vi "ROI_transform_self.vi"(6 "Color":u32[](array[colorbox])=[16860], 9 "extrinsic":cluster{"extrinsic":dbl[][], i32[]}, 10 "ROI discriptor":T2, 11 "Refnum in":T1) -> (3 "Image Out":T1)   [LabVIEW 2017]
uses:
  <vilib>/vision/Image Controls.llb/IMAQ Image.ctl
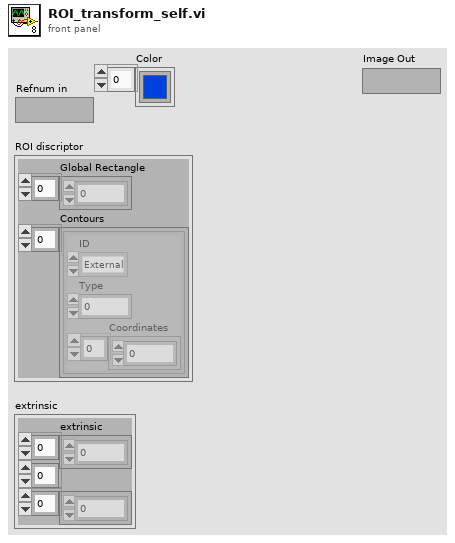
[diagram p1: front panel]
types:
  T1 = typedef "IMAQ Image.ctl" = refnum<image>
  T2 = cluster{"Global Rectangle":i32[], "Contours":cluster{"ID":enum32{"External", "Internal"}, "Type":u32, "Coordinates":i32[]}[]}
  T3 = cluster{"Start Point":cluster{"X":i32, "Y":i32}}[][]
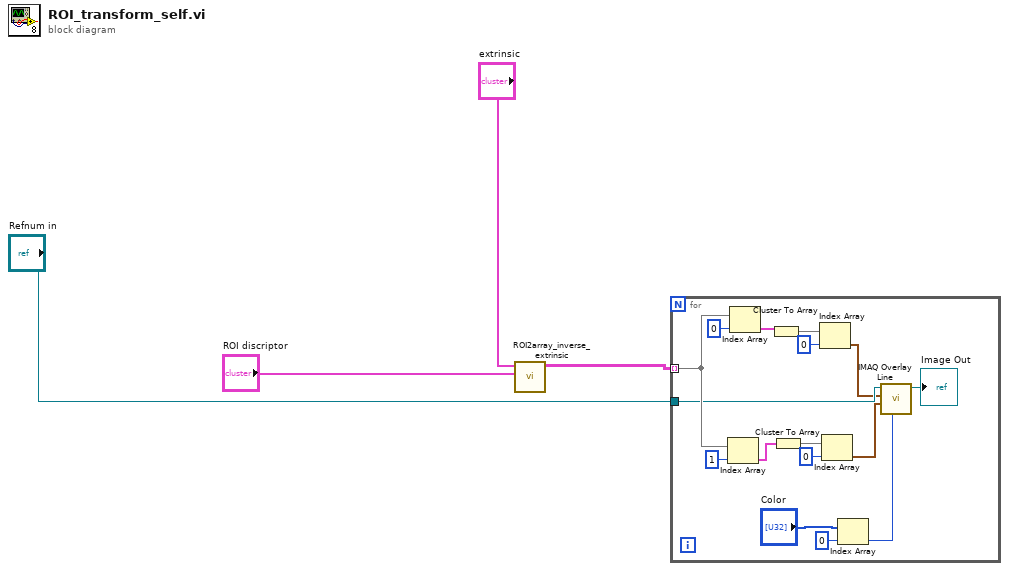
[diagram p0: block diagram]
diagram:
  n1 = call "ROI2array_inverse_extrinsic.vi"("Pad ROI 1"="ROI discriptor", "Cluster"="extrinsic") -> ("Array"=w2:T3)  [unwired: 9 in]
  n2 = for {
    tunnel: "Refnum in" -> [w14]
    tunnel: w2 -> [w19] mode=indexing
    n3 = Index Array(array=w19, index=1) -> (element=w10:cluster{"Start Point":cluster{"X":i32, "Y":i32}})
    n4 = Index Array(array=w19, index=0) -> (element=w17:cluster{"Start Point":cluster{"X":i32, "Y":i32}})
    n5 = Cluster To Array(cluster=w17) -> (array=w15:cluster{"X":i32, "Y":i32}[])
    n6 = Cluster To Array(cluster=w10) -> (array=w12:cluster{"X":i32, "Y":i32}[])
    n7 = Index Array(array=w15, index=0) -> (element=w13:cluster{"X":i32, "Y":i32})
    n8 = Index Array(array=w12, index=0) -> (element=w9:cluster{"X":i32, "Y":i32})
    n9 = Index Array(array="Color", index=0) -> (element=w5:u32)
    n10 = call "IMAQ Overlay Line"("Color"=w5, "End Point"=w9, "Start Point"=w13, "Image"=w14) -> ("Image Out"=→"Image Out":T1)  [unwired: 6 in, 1 out]
  }
